vi "MRU_Create.vi"(6 "Number to remember (10)":i32=10, 7 "CmbBox Refnum":refnum<vi>, 8 "error in (no error)":errorcluster, 9 "MRU Section Name (\"MRU\")":string="MRU", 10 "MRU INI file (c:\\mru.ini)":path=path "c:/mru.ini", 11 "reference in":refnum<class "MRU.lvclass">) -> (0 "error out":errorcluster, 3 "reference out":refnum<class "MRU.lvclass">)   [LabVIEW 2014, in "MRU.lvclass"]
doc: "Creates an MRU (Most Recently Used) Object linked to the provided Combo Box.\n\nThis class manages the contents of the Combo Box to reflect the most recently used strings. This history is stored in the INI file specified in a section named by the user, and can be updated by calling MRU_UpdateMRUList.vi.\n\nThe most common use for this Class is in an ALOHA Agent. Simply pass the Agent's Personal Data Folder INI file and a Combo Box reference to enable functionality."
uses:
  MRU.lvclass
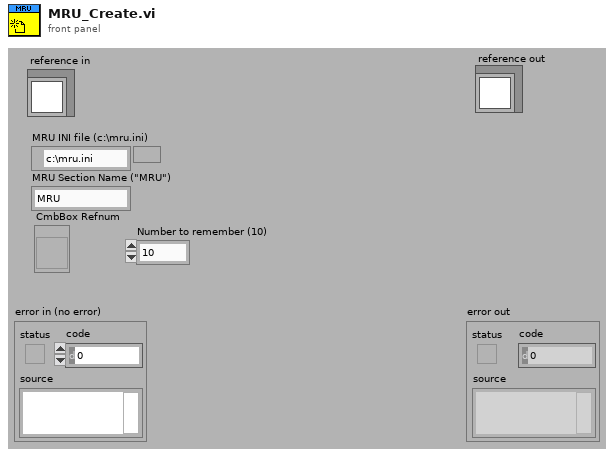
[diagram p1: front panel]
types:
  T1 = typedef "MRU.lvclass/ObjectAttributes.ctl" = cluster{"MRU INI file":path, "MRU Section Name":string, "CmbBox Refnum":refnum<vi>, "Number to remember":i32}
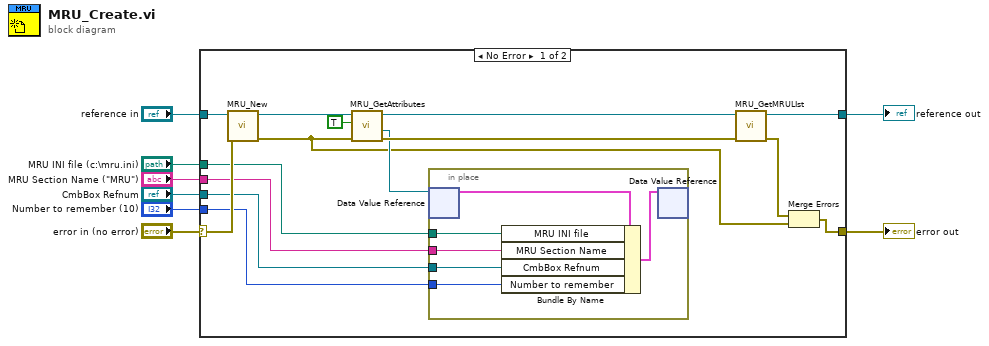
[diagram p0: block diagram]
diagram:
  n1 = case shown="No Error" "error in (no error)" {
    selector: "error in (no error)" -> [w23 w31]
    tunnel: [w20 w31] -> w8
    tunnel: "reference in" -> [w22 w30]
    tunnel: [w16 w30] -> w6
    tunnel: "MRU INI file (c:\\mru.ini)" -> [w13 _]
    tunnel: "MRU Section Name (\"MRU\")" -> [w12 _]
    tunnel: "CmbBox Refnum" -> [w11 _]
    tunnel: "Number to remember (10)" -> [w10 _]
    frame No Error {
      n2 = call "MRU_New.vi"("error in (no error)"=w23, "reference in"=w22) -> ("error out"=w9:errorcluster, "reference out"=w21:refnum<class "MRU.lvclass">)  [unwired: 2 in, 6 out]
      n3 = call "MRU_GetAttributes.vi"("error in (no error)"=w9, "OnlyGetDvrReference(False)"=TRUE, "reference in"=w21) -> ("error out"=w18:errorcluster, "DataRef"=w14:refnum<data-value>, "reference out"=w19:refnum<class "MRU.lvclass">)  [unwired: 5 in, 1 out]
      n4 = in-place {
        in-place-border: w13 -> [w28]
        in-place-border: w12 -> [w27]
        in-place-border: w11 -> [w26]
        in-place-border: w10 -> [w25]
        n5 = in-place-dvr #1(w14) -> (w29:T1)  [unwired: 1 out]
        n6 = Bundle By Name(cluster=w29, "MRU INI file"=w28, "MRU Section Name"=w27, "CmbBox Refnum"=w26, "Number to remember"=w25) -> (w24:T1)
        n7 = in-place-dvr #1(w24) -> ()  [unwired: 2 out]
      }
      n8 = call-dynamic "MRU_GetMRULIst.vi"("error in (no error)"=w18, "reference in"=w19) -> ("error out"=w17:errorcluster, "reference out"=w16:refnum<class "MRU.lvclass">)  [unwired: 8 in]
      n9 = Merge Errors(w17, w9) -> (w20:errorcluster)
    }
    frame Error {
    }
  }
  "error out" <- w8
  "reference out" <- w6
